vi "Custom_Append Front Panel Image to Report (path).vi"(0 "report in":refnum<class "NI_report.lvclass">, 1 "alignment (default)":T2, 2 "image format (jpeg)":enum32{"PNG", "JPEG", "GIF"}(ring)=enum."JPEG", 5 "VI":path, 9 "description":string, 11 "error in (no error)":errorcluster, 12 "visible area only?":bool, 13 "MS Office parameters":T1) -> (4 "report out":refnum<class "NI_report.lvclass">, 6 "VI path out":path, 8 "start out (Word)":i32, 10 "end out (Word)":i32, 15 "error out":errorcluster)   [LabVIEW 2019]
doc: "Creates an image of the front panel of the VI you specify in <B>VI</B> and appends it to a report. Wire data to the <B>VI</B> input to determine the polymorphic instance to use or manually select the instance."
uses:
  <vilib>/Utility/NIReport.llb/NI_report.lvclass
  <vilib>/Utility/NIReport.llb/HTML Report Image Alignment.ctl
  <vilib>/Utility/NIReport.llb/NI_ReportGenerationCore.lvlib
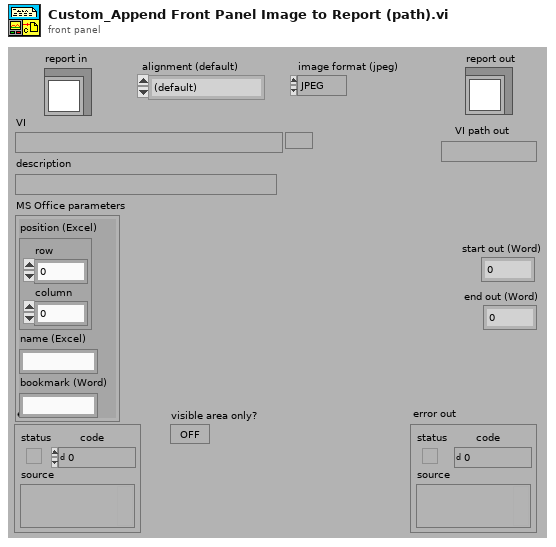
[diagram p1: front panel]
types:
  T1 = cluster{"position (Excel)":cluster{"row":i32, "column":i32}, "name (Excel)":string, "bookmark (Word)":string}
  T2 = typedef "NI_ReportGenerationCore.lvlib/HTML Report Image Alignment.ctl" = enum16{"(default)", "LEFT", "RIGHT", "TOP", "TEXTTOP", "MIDDLE", "ABSMIDDLE", "BASELINE", "BOTTOM", "ABSBOTTOM"}
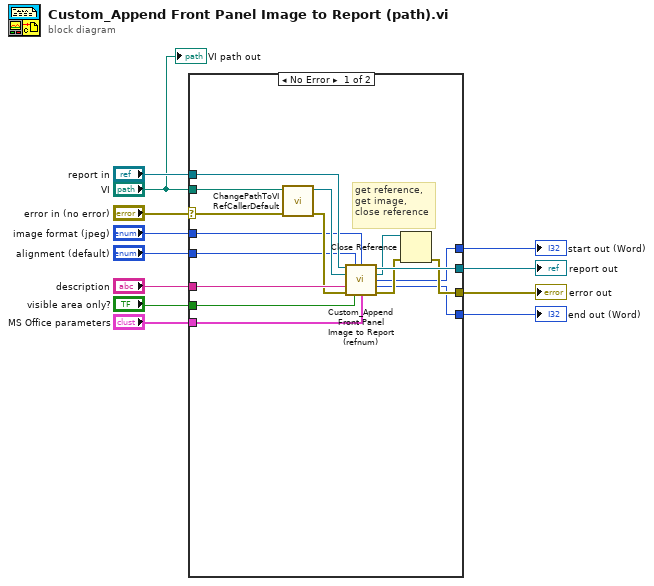
[diagram p0: block diagram]
diagram:
  n1 = case shown="No Error" "error in (no error)" {
    selector: "error in (no error)" -> [w23 w30]
    tunnel: [w16 w30] -> w11
    tunnel: "report in" -> [w27 w29]
    tunnel: "VI" -> [w13 _]
    tunnel: "description" -> [w26 _]
    tunnel: "visible area only?" -> [w24 _]
    tunnel: "alignment (default)" -> [w22 _]
    tunnel: [w21 w29] -> w5
    tunnel: "MS Office parameters" -> [w20 _]
    tunnel: "image format (jpeg)" -> [w19 _]
    tunnel: [w15 _] -> w2
    tunnel: [w14 _] -> w1
    frame No Error {
      # "get reference,\nget image,\nclose reference"
      n2 = call <vilib>:"ChangePathToVIRefCallerDefault.vi"("error in (no error)"=w23, "VI path"=w13) -> ("error out"=w25:errorcluster, "VI reference"=w28:refnum<vi>)  [unwired: 4 in]
      n3 = call "Custom_Append Front Panel Image to Report (refnum).vi"("report in"=w27, "alignment (default)"=w22, "image format (jpeg)"=w19, "VI"=w28, "description"=w26, "error in (no error)"=w25, "visible area only?"=w24, "MS Office parameters"=w20) -> ("report out"=w21:refnum<class "NI_report.lvclass">, "VI out"=w18:refnum<vi>, "start out (Word)"=w15:i32, "end out (Word)"=w14:i32, "error out"=w17:errorcluster)  [unwired: 3 in]
      n4 = Close Reference(reference=w18, error in (no error)=w17) -> (error out=w16:errorcluster)
    }
    frame Error {
    }
  }
  "error out" <- w11
  "report out" <- w5
  "start out (Word)" <- w2
  "end out (Word)" <- w1
  "VI path out" <- "VI"
